vi "ex2_producer.vi"() -> ()   [LabVIEW 2022 SP3]
uses:
  pylabview/pythonq.lvlib
  C:/Program Files (x86)/National Instruments/LabVIEW 2022/examples/Connectivity/Python/support/PythonVersionsEnum.ctl
  py_msg.ctl
panel:
  out "cur ref":string
  out "count 1":i32
  in  "wait":u32=500
  out "Wv":dbl(graph)
  in  "stop":bool
  out "count 2":i32
  out "error out":errorcluster
  # "# Created by Jeff Morgan\n# https://awakeniot.com/"
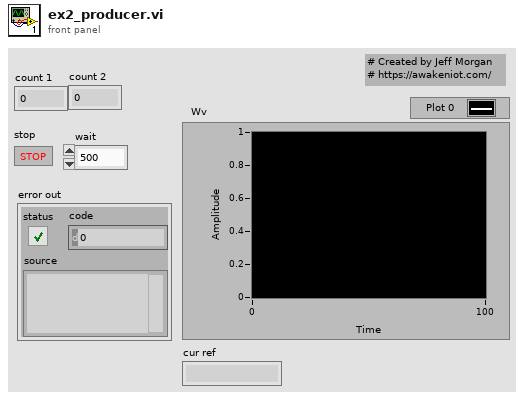
[diagram p1: front panel]
types:
  T1 = typedef "PythonVersionsEnum.ctl" = enum16{"3.6", "3.7", "3.8", "3.9"}
  T2 = typedef "pythonq.lvlib/py_cluster.ctl" = cluster{"path":path, "py":T3}
  T3 = typedef "pythonq.lvlib/py_session.ctl" = cluster{"session":refnum<k35>, "object":refnum<k38>}
  T4 = typedef "py_msg.ctl" = cluster{"double":dbl, "ref":string}
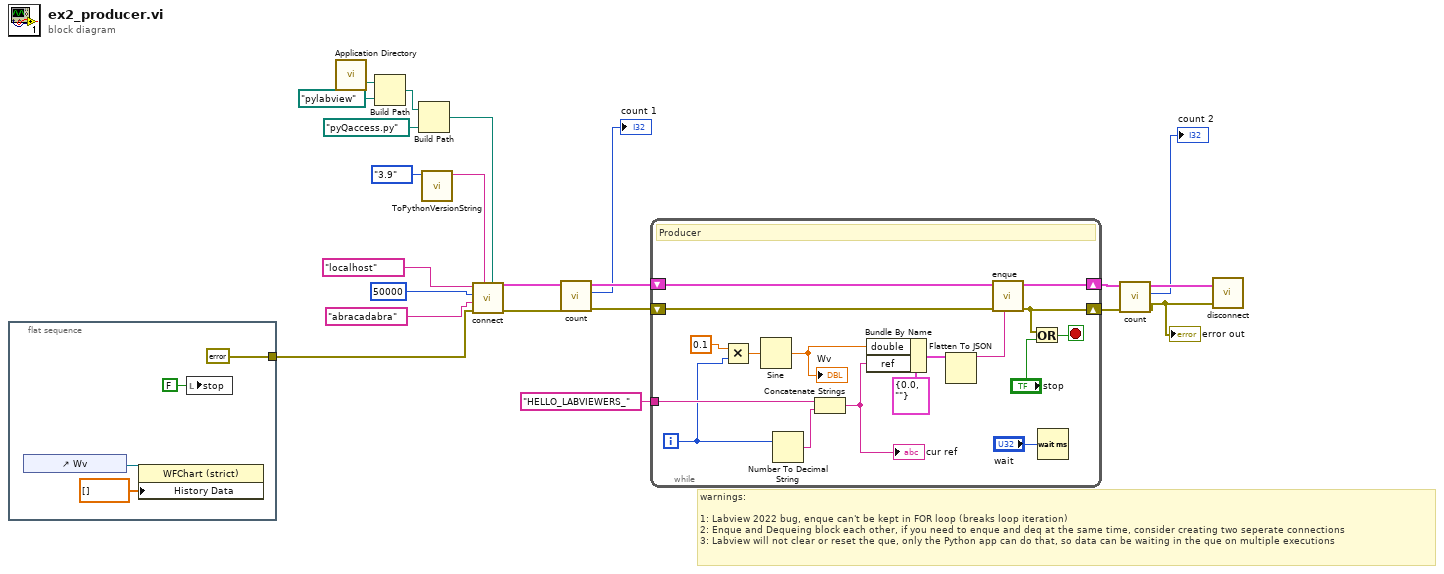
[diagram p0: block diagram]
diagram:
  # "warnings:\n\n1: Labview 2022 bug, enque can't be kept in FOR loop (breaks loop iteration)\n2: Enque and Dequeing block each other, if you need to enque and deq at the same time, consider creating two seperate connections\n3: Labview will not clear or reset the que, only the Python app can do that, so data can be waiting in the que on multiple executions"
  n1 = flat-sequence {
    tunnel: [errorcluster {"status"=FALSE, "code"=0, "source"=""} ("error in (no error)")] -> w7
    frame #0 {
      n2 = control-ref of="Wv"() -> (w24:refnum<vi>)
      n3 = property class="WFChart (strict)"(reference=w24, "History Data"=dbl[] []) -> ()  [unwired: 1 in, 2 out]
      n4 = local write "stop"(FALSE ("stop")) -> ()
    }
  }
  n5 = call <vilib>:"Application Directory.vi"() -> ("Application Directory"=w16:path)
  n6 = Build Path(base path=w16, name or relative path=path "pylabview") -> (appended path=w17:path)
  n7 = Build Path(base path=w17, name or relative path=path "pyQaccess.py") -> (appended path=w14:path)
  n8 = call "ToPythonVersionString.vi"("python version"=PythonVersionsEnum."3.9") -> ("python version string"=w19:string)  [unwired: 10 in]
  n9 = call "connect.vi"("module path"=w14, "Python version"=w19, "error in (no error)"=w7, "password"="abracadabra", "port"=50000, "ip_address"="localhost") -> ("error out"=w10:errorcluster, "py out"=w9:T2)  [unwired: 4 in]
  n10 = call "count.vi"("error in (no error)"=w10, "py in"=w9) -> ("error out"=w6:errorcluster, "count"=→"count 1":i32, "py out"=w5:T2)  [unwired: 7 in]
  n11 = while {
    shift-right: [w42] -> w4
    shift-left: w5 -> [w43]
    shift-right: [w39] -> w8
    shift-left: w6 -> [w41]
    tunnel: "HELLO_LABVIEWERS_" ("ref_prefix") -> [w36]
    i -> [w28]
    stop <- w40 stop-if-true
    # "Producer"
    n12 = Multiply(x=0.1, y=w28) -> (x*y=w30:dbl)
    n13 = Sine(x=w30) -> (sin(x)=w27:dbl)
    "Wv" <- w27
    n14 = Number To Decimal String(number=w28) -> (decimal integer string=w35:string)  [unwired: 1 in]
    n15 = Concatenate Strings(w36, w35) -> (w33:string)
    "cur ref" <- w33
    n16 = Bundle By Name(cluster=T4 {"double"=0.0, "ref"=""} ("Cluster"), "double"=w27, "ref"=w33) -> (w32:T4)
    n17 = Flatten To JSON(anything=w32) -> (JSON string=w31:string)  [unwired: 2 in, 1 out]
    n18 = call "enque.vi"("data in"=w31, "error in (no error)"=w41, "py in"=w43) -> ("error out"=w39:errorcluster, "py out"=w42:T2)  [unwired: 5 in, 2 out]
    n19 = Or(x=w39, y="stop") -> (x .or. y?=w40:bool)
    n20 = Wait (ms)(milliseconds to wait="wait") -> ()  [unwired: 1 out]
  }
  n21 = call "count.vi"("error in (no error)"=w8, "py in"=w4) -> ("error out"=w2:errorcluster, "count"=→"count 2":i32, "py out"=w12:T2)  [unwired: 7 in]
  "error out" <- w2
  n22 = call "disconnect.vi"("error in (no error)"=w2, "py in"=w12) -> ()  [unwired: 9 in, 1 out]
